vi "Init.vi"(8 "error in (no error)":errorcluster, 10 "Application Ref":refnum<class "Message Enqueuer.lvclass">) -> (0 "error out":errorcluster, 3 "AutomationContext out":refnum<class "AutomationContext.lvclass">)   [LabVIEW 2023, in "Automation.lvlib" / "AutomationContext.lvclass"]
uses:
  AutomationContext.lvclass
  <vilib>/ActorFramework/Message Enqueuer/Message Enqueuer.lvclass
  AutomationContext.lvclass/AutomationContext.ctl
panel:
  in  "AutomationContext in":refnum<class "AutomationContext.lvclass">
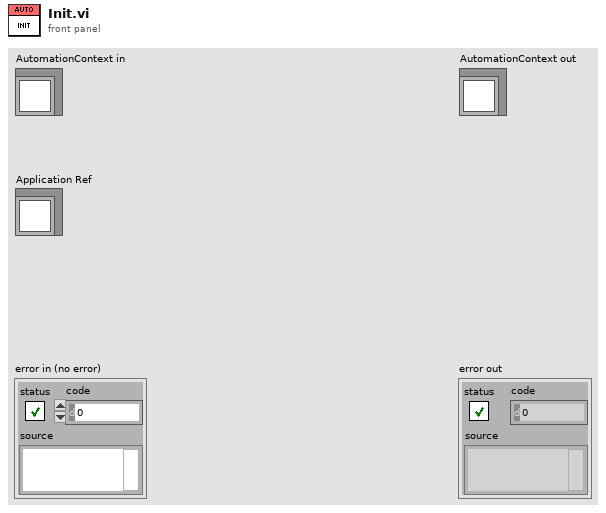
[diagram p1: front panel]
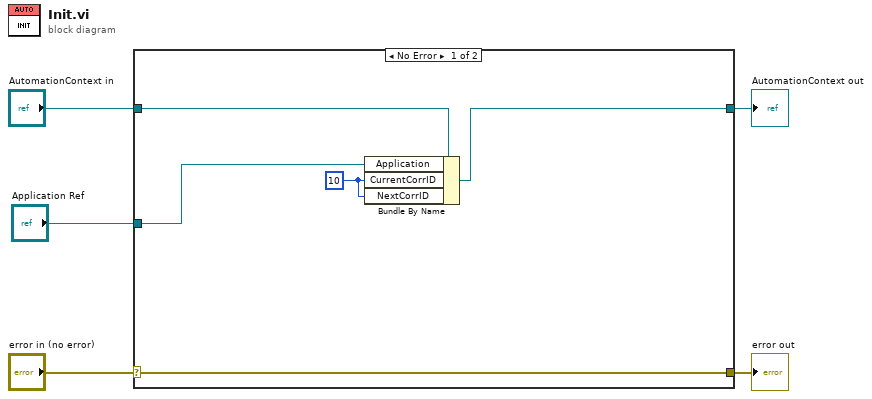
[diagram p0: block diagram]
diagram:
  n1 = case shown="No Error" "error in (no error)" {
    selector: "error in (no error)" -> [w10 w12]
    tunnel: [w10 w12] -> w4
    tunnel: [w8 w11] -> w2
    tunnel: "AutomationContext in" -> [w9 w11]
    tunnel: "Application Ref" -> [w7 _]
    frame No Error {
      w6 = u32 10 ("Correlation ID")
      n2 = Bundle By Name(cluster=w9, "Application"=w7, "CurrentCorrID"=w6, "NextCorrID"=w6) -> (w8:refnum<class "AutomationContext.lvclass">)
    }
    frame Error {
    }
  }
  "error out" <- w4
  "AutomationContext out" <- w2
